vi "rethinkdb_tcp_parse_error_json.vi"(8 "error in (no error)":errorcluster, 11 "message":string) -> (0 "error out":errorcluster, 1 "is error?":bool)   [LabVIEW 2017]
uses:
  cabca6b0-f2c7-43cf-a6e5-c7a1e05d8cdf.vi
  json/rethinkdb_json_to_cluster.vi
  json/rethinkdb_json_type_cast.vi
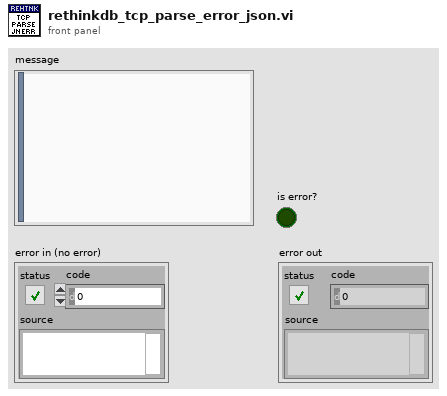
[diagram p1: front panel]
types:
  T1 = cluster{"error_code":i32, "error":string, "success":bool}
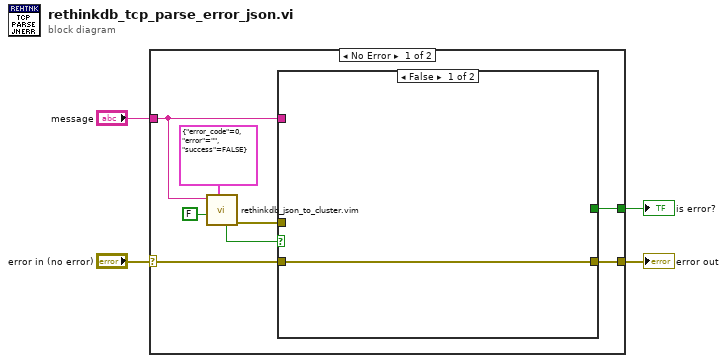
[diagram p0: block diagram]
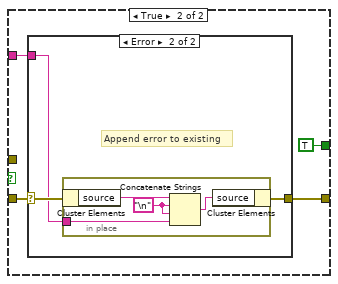
[diagram p2: hidden frame]
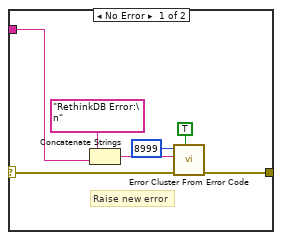
[diagram p3: hidden frame]
diagram:
  n1 = case shown="No Error" "error in (no error)" {
    selector: "error in (no error)" -> [w6 w32]
    tunnel: [w12 w32] -> w4
    tunnel: [w11 _] -> w3
    tunnel: "message" -> [w8 _]
    frame No Error {
      n2 = call "rethinkdb_json_to_cluster.vim"("type"=T1 {"error_code"=0, "error"="", "success"=FALSE} ("handshake"), "allow missing? (F)"=FALSE, "json"=w8) -> ("error out"=w5:errorcluster, "complete match?"=w7:bool)  [unwired: 5 in, 2 out]
      n3 = case shown="False" w7 {
        tunnel: w6 -> [w13 w17]
        tunnel: w8 -> [_ w15]
        tunnel: [w13 w16] -> w12
        tunnel: [_ TRUE] -> w11
        tunnel: w5 -> [_ _]
        frame False {
        }
        frame True {
          n4 = case shown="Error" w17 {
            selector: w17 -> [w24 w27]
            tunnel: [w21 w26] -> w16
            tunnel: w15 -> [w19 w25]
            frame No Error {
              # "Raise new error"
              n5 = Concatenate Strings("RethinkDB Error:\n" ("error message (\"\")"), w19) -> (w18:string)
              n6 = call <vilib>:"Error Cluster From Error Code.vi"("show call chain? (False)"=TRUE, "error in (no error)"=w24, "error message (\"\")"=w18, "error code (0)"=8999) -> ("error out"=w21:errorcluster)  [unwired: 5 in]
            }
            frame Error {
              # "Append error to existing"
              n7 = in-place {
                in-place-border: w25 -> [w29]
                w28 = "\n"
                n8 = in-place-cluster #1(w27) -> ("source"=w31:string)
                n9 = Concatenate Strings(w31, w28, w28, w29) -> (w30:string)
                n10 = in-place-cluster #1("source"=w30) -> (w26:errorcluster)
              }
            }
          }
        }
      }
    }
    frame Error {
    }
  }
  "error out" <- w4
  "is error?" <- w3
